vi "save to common.vi"(9 "Messages read 3":T1, 10 "Common messages":path) -> ()   [LabVIEW 2015, in "Biblioteka moduł map v3.lvlib" / "task erl.lvlib"]
uses:
  TASK ERL/task erl.lvlib
  KML/KML.lvlib
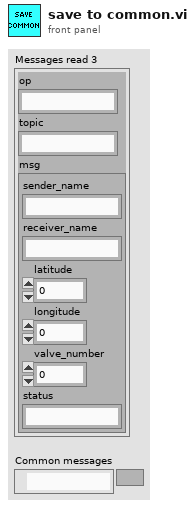
[diagram p1: front panel]
types:
  T1 = cluster{"op":string, "topic":string, "msg":cluster{"sender_name":string, "receiver_name":string, "latitude":dbl, "longitude":dbl, "valve_number":i32, "status":string}}
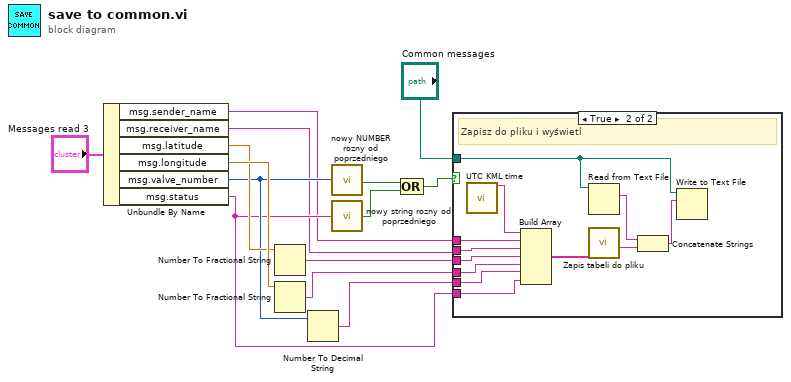
[diagram p0: block diagram]
diagram:
  n1 = Unbundle By Name("Messages read 3") -> ("msg.sender_name"=w6:string, "msg.receiver_name"=w7:string, "msg.latitude"=w11:dbl, "msg.longitude"=w14:dbl, "msg.valve_number"=w9:i32, "msg.status"=w8:string)
  n2 = Number To Fractional String(number=w11) -> (F-format string=w12:string)  [unwired: 3 in]
  n3 = Number To Fractional String(number=w14) -> (F-format string=w13:string)  [unwired: 3 in]
  n4 = Number To Decimal String(number=w9) -> (decimal integer string=w10:string)  [unwired: 1 in]
  n5 = call "nowy NUMBER rozny od poprzedniego.vi"("Numeric"=w9) -> ("x != y?"=w1:bool)  [unwired: 4 in]
  n6 = call "nowy string rozny od poprzedniego.vi"("String"=w8) -> ("x != y?"=w2:bool)  [unwired: 4 in]
  n7 = Compound Arithmetic op=OR(w1, w2) -> (w3:bool)
  n8 = case shown="True" w3 {
    tunnel: "Common messages" -> [_ w24]
    tunnel: w6 -> [_ w21]
    tunnel: w7 -> [_ w20]
    tunnel: w8 -> [_ w19]
    tunnel: w10 -> [_ w17]
    tunnel: w12 -> [_ w16]
    tunnel: w13 -> [_ w15]
    frame False {
      # "nic nie rob"
    }
    frame True {
      # "Zapisz do pliku i wyświetl"
      n9 = call "UTC KML time.vi"() -> ("String"=w22:string)  [unwired: 19 in]
      n10 = Build Array(w22, w21, w20, w16, w15, w17, w19) -> (w23:string[])
      n11 = Read from Text File(file (use dialog)=w24) -> (text=w18:string)  [unwired: 3 in, 3 out]
      n12 = call "Zapis tabeli do pliku.vi"("1d array in"=w23) -> ("for 1d array out"=w25:string)  [unwired: 7 in, 1 out]
      n13 = Concatenate Strings(w18, w25) -> (w26:string)
      n14 = Write to Text File(file (use dialog)=w24, text=w26) -> ()  [unwired: 2 in, 3 out]
    }
  }
